vi "Build File Name.vi"(0 "Folder":path caption="Ausgewählter Pfad", 1 "Extension":string) -> (4 "Path Out":path, 5 "File Path":path, 6 "File Path String":string, 7 "Error":errorcluster)   [LabVIEW 2010]
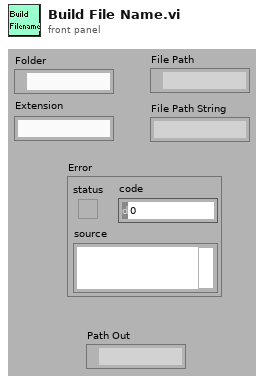
[diagram p1: front panel]
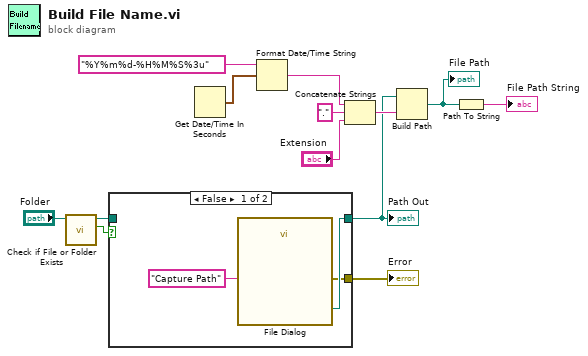
[diagram p0: block diagram]
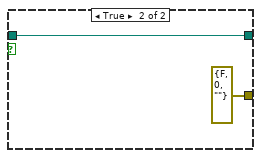
[diagram p2: hidden frame]
diagram:
  n1 = call <vilib>:"Check if File or Folder Exists.vi"("path"="Folder") -> ("file or folder exists?"=w5:bool, "dup path"=w3:path)  [unwired: 8 in, 1 out]
  n2 = case shown="False" w5 {
    tunnel: [w15 w18] -> w1
    tunnel: w3 -> [_ w18]
    tunnel: [w14 errorcluster {"status"=FALSE, "code"=0, "source"=""} ("error out")] -> w2
    frame False {
      n3 = call "File Dialog"("prompt"="Capture Path" ("pattern label")) -> ("selected path"=w15:path, "error out"=w14:errorcluster)  [unwired: 11 in, 2 out]
    }
    frame True {
    }
  }
  "Error" <- w2
  "Path Out" <- w1
  n4 = Get Date/Time In Seconds() -> (seconds since 1Jan1904=w13:timestamp)
  n5 = Format Date/Time String(time format string (%c)="%Y%m%d-%H%M%S%3u", seconds (now)=w13) -> (date/time string=w9:string)  [unwired: 1 in]
  n6 = Concatenate Strings(w9, "." ("string"), "Extension") -> (w8:string)
  n7 = Build Path(base path=w1, name or relative path=w8) -> (appended path=w7:path)
  "File Path" <- w7
  n8 = Path To String(path=w7) -> (string=→"File Path String":string)
